vi "CCM-Show Table.vi"(0 "Table":T1[](array[typedef]), 5 "Required":string[](array[string]), 7 "Table Ref":refnum<vi>, 9 "List Ref":refnum<vi>, 11 "Force required":bool) -> ()   [LabVIEW 2020]
uses:
  Type Defs/CM-Connection.ctl
  Utility VIs/Controls/KTable/KTable.xctl
  Utility VIs/Controls/KListboxEx/KListboxEx.xctl
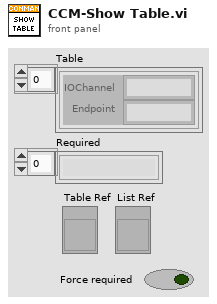
[diagram p1: front panel]
types:
  T1 = typedef "CM-Connection.ctl" = cluster{"IOChannel":string, "Endpoint":string}
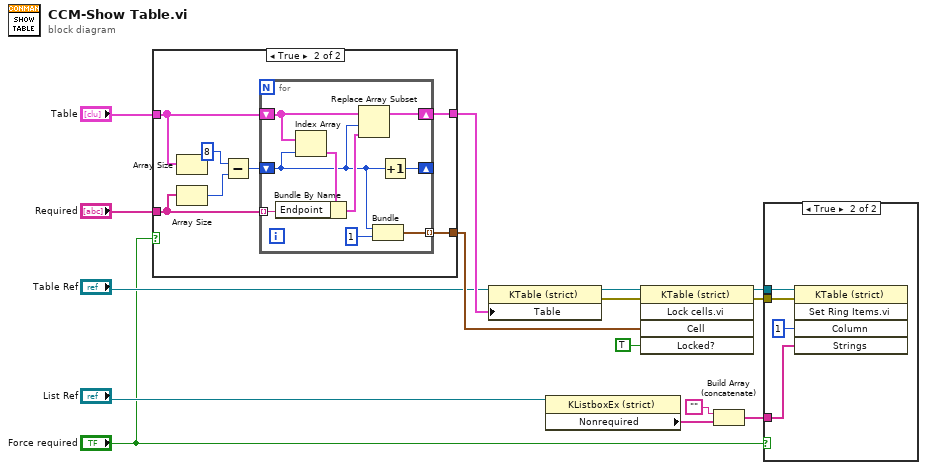
[diagram p0: block diagram]
diagram:
  n1 = case shown="True" "Force required" {
    tunnel: "Required" -> [_ w19]
    tunnel: "Table" -> [w16 w23]
    tunnel: [w16 w21] -> w15
    tunnel: [_ w20] -> w12
    frame False {
    }
    frame True {
      n2 = Array Size(array=w23) -> ()  [unwired: 1 out]
      n3 = Array Size(array=w19) -> (size(s)=w18:i32)
      n4 = Subtract(x=8, y=w18) -> (x-y=w22:i32)
      n5 = for {
        tunnel: w19 -> [w31] mode=indexing
        shift-right: [w27] -> w21
        shift-left: w23 -> [w30]
        shift-right: [w28] -> _
        shift-left: w22 -> [w25]
        tunnel: [w24] -> w20 mode=indexing
        n6 = Index Array(array=w30, index=w25) -> (element=w32:T1)
        n7 = Bundle By Name(cluster=w32, "Endpoint"=w31) -> (w29:T1)
        n8 = Replace Array Subset(array=w30, new element=w29, index=w25) -> (w27:T1[])
        n9 = Bundle(w25, 1) -> (w24:cluster{i32, i32})  [unwired: 1 in]
        n10 = Increment(x=w25) -> (x+1=w28:i32)
      }
    }
  }
  n11 = property on="Property Node" class="KTable (strict)"(reference="Table Ref", "Table"=w15) -> (reference out=w14:refnum<vi>, error out=w13:errorcluster)  [unwired: 1 in]
  n12 = property class="KListboxEx (strict)"(reference="List Ref") -> ("Nonrequired"=w9:string[])  [unwired: 1 in, 2 out]
  n13 = invoke class="KTable (strict)" method="Lock cells.vi"(reference=w14, error in=w13, "Cell"=w12, "Locked?"=TRUE) -> (reference out=w11:refnum<vi>, error out=w10:errorcluster)  [unwired: 1 in, 3 out]
  n14 = Build Array (concatenate)("", w9) -> (w8:string[])
  n15 = case shown="True" "Force required" {
    tunnel: w11 -> [_ w35]
    tunnel: w10 -> [_ w36]
    tunnel: w8 -> [_ w34]
    frame False {
    }
    frame True {
      n16 = invoke class="KTable (strict)" method="Set Ring Items.vi"(reference=w35, error in=w36, "Column"=1, "Strings"=w34) -> ()  [unwired: 1 in, 5 out]
    }
  }
